vi "HW.FlocEnd Mockup.vi"() -> ()   [LabVIEW 2015, in "AguaClara Library.lvlib"]
uses:
  AguaClara Library.lvlib
  toolbar icons/help.ctl
  <vilib>/Platform/browser.llb/Open URL in Default Browser (string).vi
panel:
  in  "URL":string="https://confluence.cornell.edu/display/AGUACLARA/AguaClara+Design+Tool"
  in  "Help Button":T1
  in  "Tab Control":enum32{"Page 1", "Page 2"}(tab)
  in  "write":bool
  in  "Floc tank depth controls":T2={"HW.FlocEnd"=enum."User specified depth", "HW.FlocEndDepth"=2.0} {"HW.FlocEndDepth" min=0.5 max=5.0 step=0.01 format="%.2f"}
  out "HW.FlocEndControl":dbl[unit]
  in  "HW.FlocEnd Input":dbl[unit]
  in  "read Button":bool
  in  "stop":bool
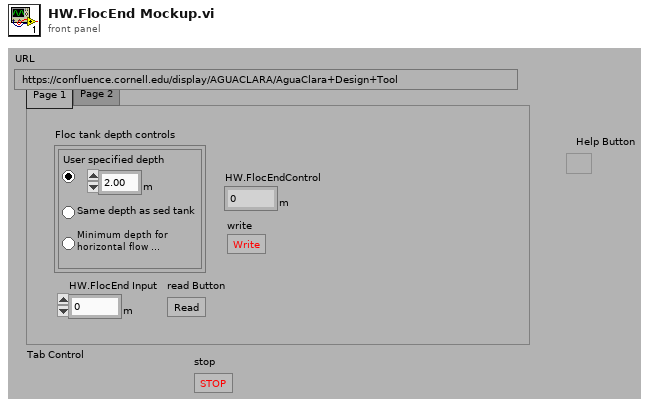
[diagram p1: front panel]
types:
  T1 = typedef "help.ctl" = bool
  T2 = cluster{"HW.FlocEnd":enum32{"User specified depth", "Same depth as sed tank", "Minimum depth for horizontal flow FLocculator"}, "HW.FlocEndDepth":dbl[unit]}
  T3 = enum32{"User specified depth", "Same depth as sed tank", "Minimum depth for horizontal flow FLocculator"}
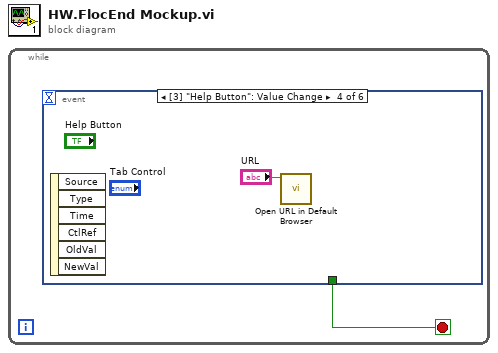
[diagram p0: block diagram]
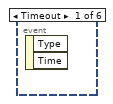
[diagram p2: hidden frame]
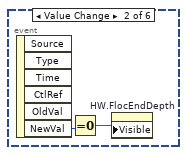
[diagram p3: hidden frame]
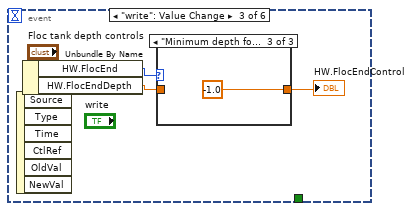
[diagram p4: hidden frame]
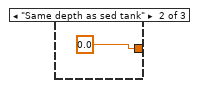
[diagram p6: hidden frame]
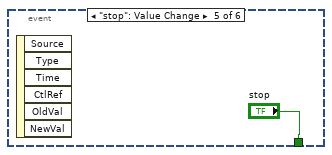
[diagram p7: hidden frame]
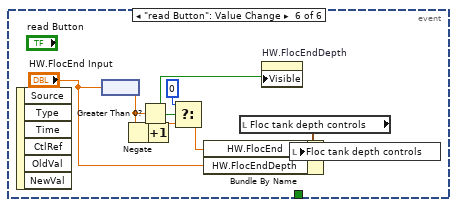
[diagram p8: hidden frame]
diagram:
  n1 = while {
    stop <- w1 stop-if-true
    n2 = event shown="[3] \"Help Button\": Value Change" {
      selector: _ -> [_ _ _ _ _ _]
      dyn-events: _ -> [_ _ _ _ _ _]
      timeout: _ -> [_ _ _ _ _ _]
      tunnel: [_ _ _ _ "stop" _] -> w1
      event Timeout {
        n3 = event-data() -> ()  [unwired: 1 in, 2 out]
      }
      event "Floc tank depth controls.HW.FlocEnd": Value Change {
        n4 = event-data() -> ("NewVal"=w3:T3)  [unwired: 1 in, 5 out]
        n5 = Equal To 0?(x=w3) -> (x = 0?=w2:bool)
        n6 = property on="HW.FlocEndDepth" class="DigNum (strict)"("Visible"=w2) -> ()  [unwired: 2 in, 2 out]
      }
      event "write": Value Change {
        n7 = event-data() -> ()  [unwired: 1 in, 6 out]
        n8 = Unbundle By Name("Floc tank depth controls") -> ("HW.FlocEnd"=w6:T3, "HW.FlocEndDepth"=w5:dbl[unit])
        n9 = case shown="\"Minimum depth for horizontal flow FLocculator\"" w6 {
          tunnel: [w8 dbl[unit] 0.0 ("HW.FlocEndControl") dbl[unit] -1.0 ("HW.FlocEndControl")] -> w4
          tunnel: w5 -> [w8 _ _]
          frame "User specified depth", Default {
          }
          frame "Same depth as sed tank" {
          }
          frame "Minimum depth for horizontal flow FLocculator" {
          }
        }
        "HW.FlocEndControl" <- w4
      }
      event Value Change {
        n10 = event-data() -> ()  [unwired: 1 in, 6 out]
        n11 = call-poly <vilib>:"Open URL in Default Browser.vi"("URL"="URL") -> ()  [unwired: 5 in, 2 out]
      }
      event "stop": Value Change {
        n12 = event-data() -> ()  [unwired: 1 in, 6 out]
      }
      event "read Button": Value Change {
        n13 = event-data() -> ()  [unwired: 1 in, 6 out]
        n14 = node("HW.FlocEnd Input") -> (w17:dbl)
        n15 = Negate(x=w17) -> (-x=w14:dbl)
        n16 = Greater Than 0?(x=w17) -> (x > 0?=w15:bool)
        n17 = Increment(x=w14) -> (x+1=w13:dbl)
        n18 = Select(t=0, s=w15, f=w13) -> (s? t:f=w16:dbl)
        n19 = local read "Floc tank depth controls"() -> (w21:T2)
        n20 = Bundle By Name(cluster=w21, "HW.FlocEnd"=w16, "HW.FlocEndDepth"="HW.FlocEnd Input") -> (w20:T2)
        n21 = property on="HW.FlocEndDepth" class="DigNum (strict)"("Visible"=w15) -> ()  [unwired: 2 in, 2 out]
        n22 = local write "Floc tank depth controls"(w20) -> ()
      }
    }
  }
